vi "MultiTaskElasticNet.vi"(8 "error in":errorcluster) -> (0 "error out":errorcluster, 3 "out":refnum<class "MultiTaskElasticNet.lvclass">)   [LabVIEW 2020]
doc: "Multi-task ElasticNet model trained with L1/L2 mixed-norm as\n regularizer.\n\n The optimization objective for MultiTaskElasticNet is::\n\n (1 / (2 * n_samples)) * ||Y - XW||_Fro^2\n + alpha * l1_ratio * ||W||_21\n + 0.5 * alpha * (1 - l1_ratio) * ||W||_Fro^2\n\n Where::\n\n ||W||_21 = sum_i sqrt(sum_j W_ij ^ 2)\n\n i.e. the sum of norms of each row.\n\n Read more in the :ref:`User Guide <multi_task_elastic_net>`.\n\n Parameters\n ----------\n alpha : float, default=1.0\n Constant that multiplies the L1/L2 term. Defaults to 1.0.\n\n l1_ratio : float, default=0.5\n The ElasticNet mixing parameter, with 0 < l1_ratio <= 1.\n For l1_ratio = 1 the penalty is an L1/L2 penalty. For l1_ratio = 0 it\n is an L2 penalty.\n For ``0 < l1_ratio < 1``, the penalty is a combination of L1/L2 and L2.\n\n fit_intercept : bool, default=True\n Whether to calculate the intercept for this model. If set\n to false, no intercept will be used in calculations\n (i.e. data is expected to be centered).\n\n normalize : bool, default=False\n This parameter is ignored when ``fit_intercept`` is set to False.\n If True, the regressors X will be normalized before regression by\n subtracting the mean and dividing by the l2-norm.\n If you wish to standardize, please use\n :class:`~sklearn.preprocessing.StandardScaler` before calling ``fit``\n on an estimator with ``normalize=False``.\n\n copy_X : bool, default=True\n If ``True``, X will be copied; else, it may be overwritten.\n\n max_iter : int, default=1000\n The maximum number of iterations.\n\n tol : float, default=1e-4\n The tolerance for the optimization: if the updates are\n smaller than ``tol``, the optimization code checks the\n dual gap for optimality and continues until it is smaller\n than ``tol``.\n\n warm_start : bool, default=False\n When set to ``True``, reuse the solution of the previous call to fit as\n initialization, otherwise, just erase the previous solution.\n See :term:`the Glossary <warm_start>`.\n\n random_state : int, RandomState instance, default=None\n The seed of the pseudo random number generator that selects a random\n feature to update. Used when ``selection`` == 'random'.\n Pass an int for reproducible output across multiple function calls.\n See :term:`Glossary <random_state>`.\n\n selection : {'cyclic', 'random'}, default='cyclic'\n If set to 'random', a random coefficient is updated every iteration\n rather than looping over features sequentially by default. This\n (setting to 'random') often leads to significantly faster convergence\n especially when tol is higher than 1e-4.\n\n Attributes\n ----------\n intercept_ : ndarray of shape (n_tasks,)\n Independent term in decision function.\n\n coef_ : ndarray of shape (n_tasks, n_features)\n Parameter vector (W in the cost function formula). If a 1D y is\n passed in at fit (non multi-task usage), ``coef_`` is then a 1D array.\n Note that ``coef_`` stores the transpose of ``W``, ``W.T``.\n\n n_iter_ : int\n Number of iterations run by the coordinate descent solver to reach\n the specified tolerance.\n\n dual_gap_ : float\n The dual gaps at the end of the optimization.\n\n eps_ : float\n The tolerance scaled scaled by the variance of the target `y`.\n\n sparse_coef_ : sparse matrix of shape (n_features,) or (n_tasks, n_features)\n Sparse representation of the `coef_`.\n\n \nAvailable methods:\nGet Attributes\nGet Params\nSet Params"
uses:
  MultiTaskElasticNet.lvclass
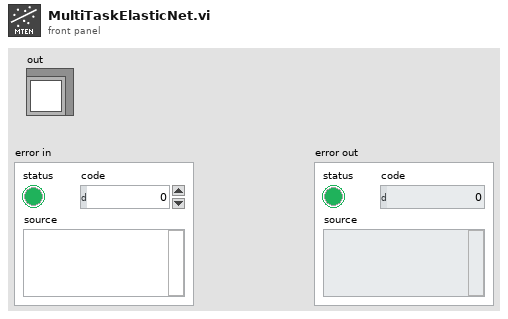
[diagram p1: front panel]
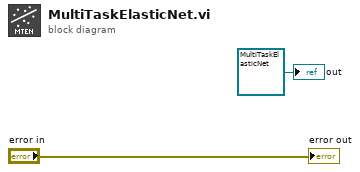
[diagram p0: block diagram]
diagram:
  "out" <- refnum<class "MultiTaskElasticNet.lvclass"> refnum ("model")
  "error out" <- "error in"
